vi "APC_HRL.vi"(0 "Pcyl":dbl[][](array[numeric])=array1x7200[7200 elements], 1 "exhaust pressure":dbl[][](array[numeric])=array1x7200[7200 elements], 2 "FilterCoefs":T3={"IIR LowPass"={"filter structure"=enum."IIR 2nd Order", "Reverse Coefficients"=[-1.7786317778245848, 0.8008026466657077], "Forward Coefficients"=[0.005542717210280682, 0.011085434420561363, 0.005542717210280682]}, "IIR HighPass"={"filter structure"=enum."IIR 2nd Order", "Reverse Coefficients"=[], "Forward Coefficients"=[]}} {"IIR LowPass"."Forward Coefficients" format="%.4f"; "IIR LowPass"."Reverse Coefficients" format="%.4f"}, 3 "Expected IMEP":dbl) -> (4 "LPfilt Pcyl":dbl[][](array[numeric]), 5 "HRL [J]":dbl[][](array[numeric]), 6 "CombustionAnalysisCluster":T2={"IMEPn [bar]"=[nan, nan, nan, nan, nan, nan], "IMEPg [bar]"=[nan, nan, nan, nan, nan, nan], "MAPO [bar/CAD]"=[nan, nan, nan, nan, nan, nan], "maxQ [J]"=[nan, nan, nan, nan, nan, nan], "CA10  [CADATDC]"=[nan, nan, nan, nan, nan, nan], "CA50 [CADATDC]"=[nan, nan, nan, nan, nan, nan], "CA90 [CADATDC]"=[nan, nan, nan, nan, nan, nan], "Pmax [bar]"=[nan, nan, nan, nan, nan, nan], "IMEPstd [bar]"=[nan, nan, nan, nan, nan, nan], "CA03  [CADATDC]"=[nan, nan, nan, nan, nan, nan], "CA97  [CADATDC]"=[nan, nan, nan, nan, nan, nan], "CA10CA90 [CADATDC]"=[nan, nan, nan, nan, nan, nan], "maxdpdCAD [bar/CAD]"=[nan, nan, nan, nan, nan, nan], "kappa_comp [-]"=[nan, nan, nan, nan, nan, nan], "kappa_exp [-]"=[nan, nan, nan, nan, nan, nan], "PMEP [bar]"=[nan, nan, nan, nan, nan, nan], "RI [-]"=[nan, nan, nan, nan, nan, nan]}, 7 "HPfilt Pcyl":dbl[][](array[numeric]), 8 "PcylDiagWarningsAndErrors":T1[](array[typedef]))   [LabVIEW 2020]
uses:
  controls/APC_CombustionMetrics.ctl
  controls/APC_PcylDiag.ctl
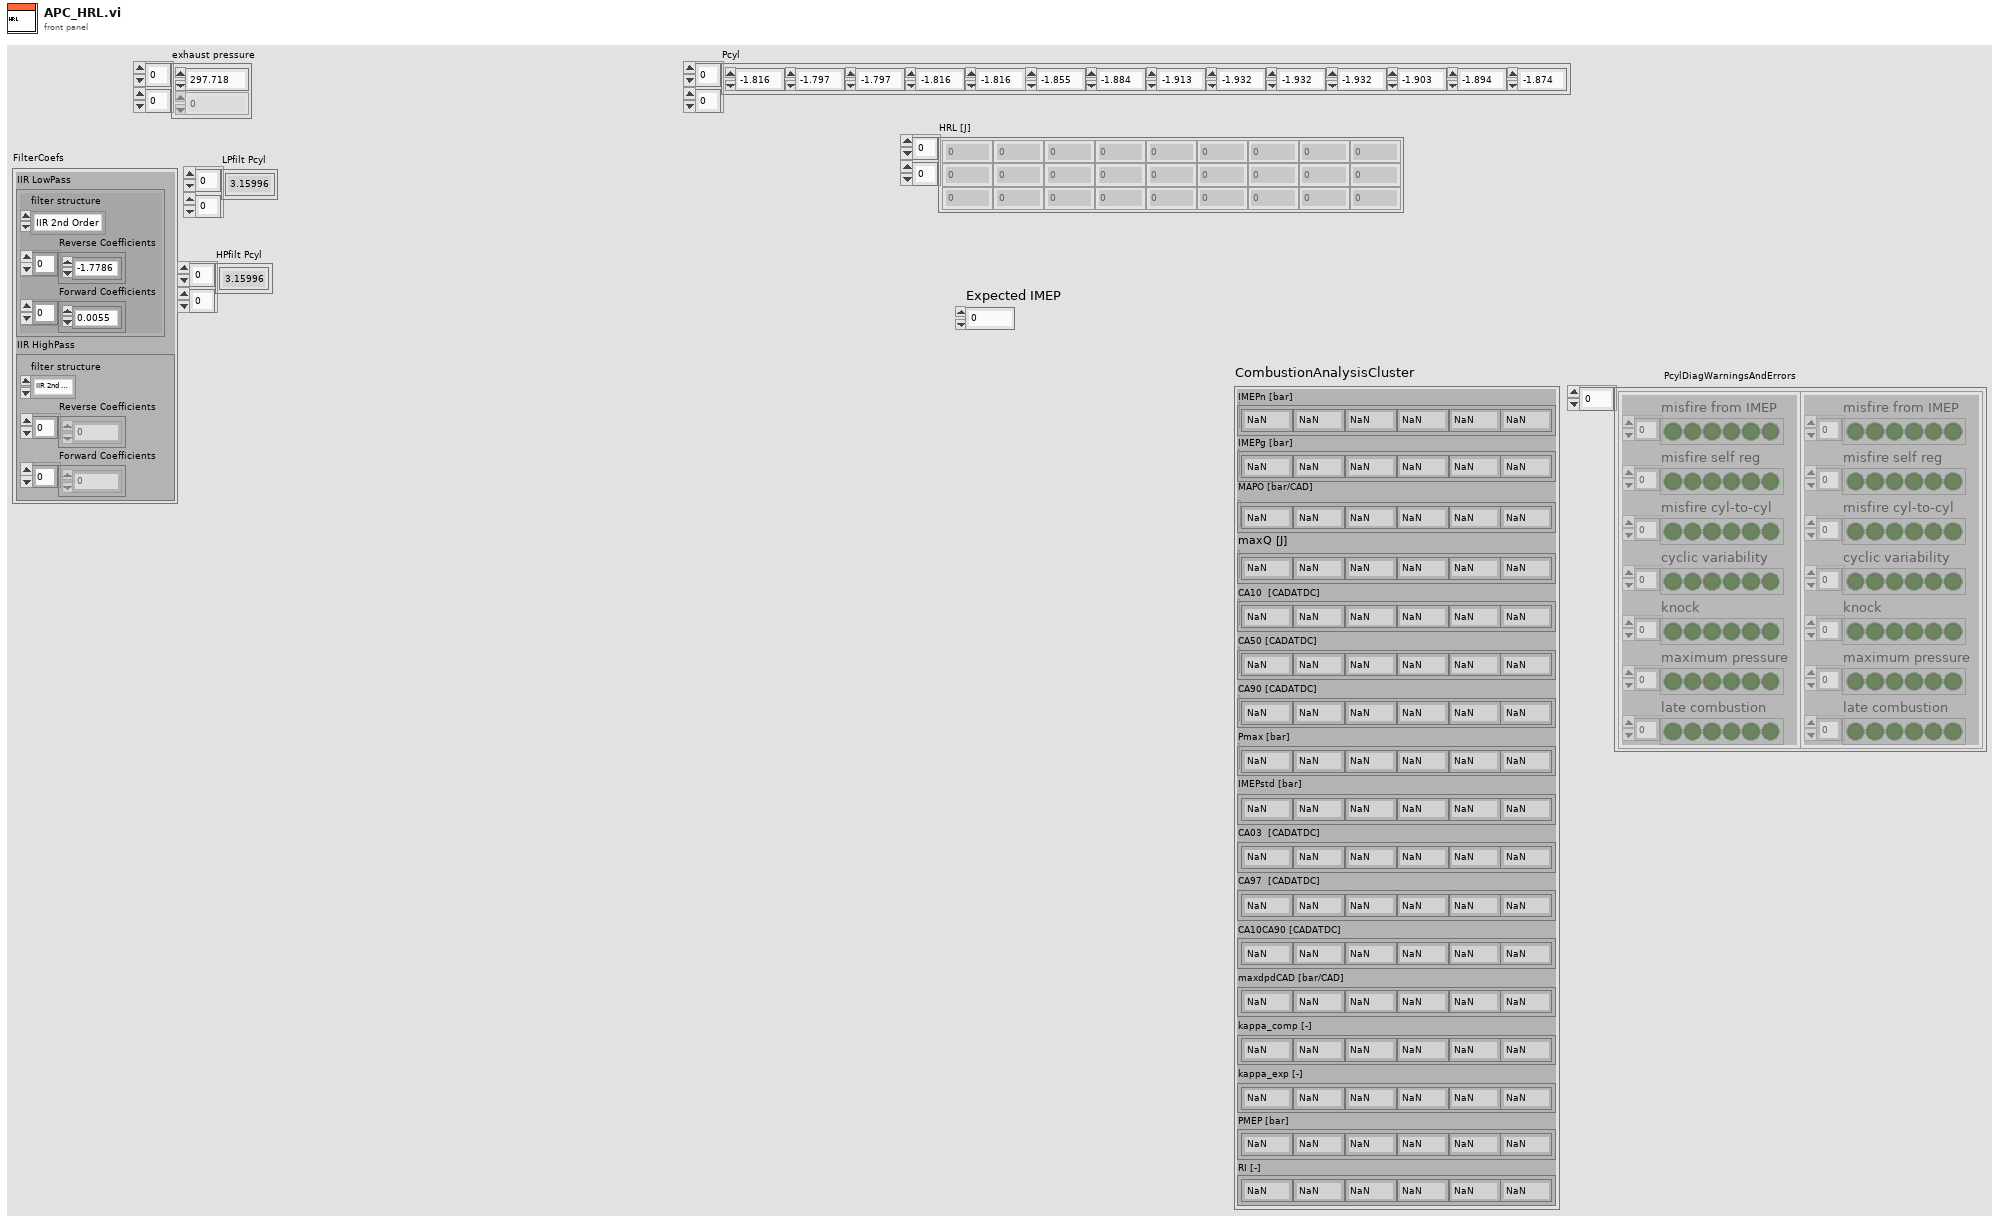
[diagram p1: front panel]
types:
  T1 = typedef "APC_PcylDiag.ctl" = cluster{"misfire from IMEP":bool[], "misfire self reg":bool[], "misfire cyl-to-cyl":bool[], "cyclic variability":bool[], "knock":bool[], "maximum pressure":bool[], "late combustion":bool[]}
  T2 = typedef "APC_CombustionMetrics.ctl" = cluster{"IMEPn [bar]":dbl[], "IMEPg [bar]":dbl[], "MAPO [bar/CAD]":dbl[], "maxQ [J]":dbl[], "CA10  [CADATDC]":dbl[], "CA50 [CADATDC]":dbl[], "CA90 [CADATDC]":dbl[], "Pmax [bar]":dbl[], "IMEPstd [bar]":dbl[], "CA03  [CADATDC]":dbl[], "CA97  [CADATDC]":dbl[], "CA10CA90 [CADATDC]":dbl[], "maxdpdCAD [bar/CAD]":dbl[], "kappa_comp [-]":dbl[], "kappa_exp [-]":dbl[], "PMEP [bar]":dbl[], "RI [-]":dbl[]}
  T3 = cluster{"IIR LowPass":cluster{"filter structure":enum32{"IIR 2nd Order", "IIR 4th Order"}, "Reverse Coefficients":dbl[], "Forward Coefficients":dbl[]}, "IIR HighPass":cluster{"filter structure":enum32{"IIR 2nd Order", "IIR 4th Order"}, "Reverse Coefficients":dbl[], "Forward Coefficients":dbl[]}}
  T4 = cluster{"filter structure":enum32{"IIR 2nd Order", "IIR 4th Order"}, "Reverse Coefficients":dbl[], "Forward Coefficients":dbl[]}
  T5 = typedef "APC_volume.ctl" = cluster{"V [m^3]":dbl[], "dV [m^3/CAD]":dbl[], "Vdis [m^3]":dbl, "Surface [m^2]":dbl[], "CAD/sample":dbl}
  T6 = typedef "APC_CylMetrics.ctl" = cluster{"maxdPdCAD [bar/CAD]":dbl, "kappa_comp":dbl, "kappa_exp":dbl, "maxQ [J]":dbl, "CA03":dbl, "CA10":dbl, "CA50":dbl, "CA90":dbl, "CA97":dbl, "CA10CA90":dbl}
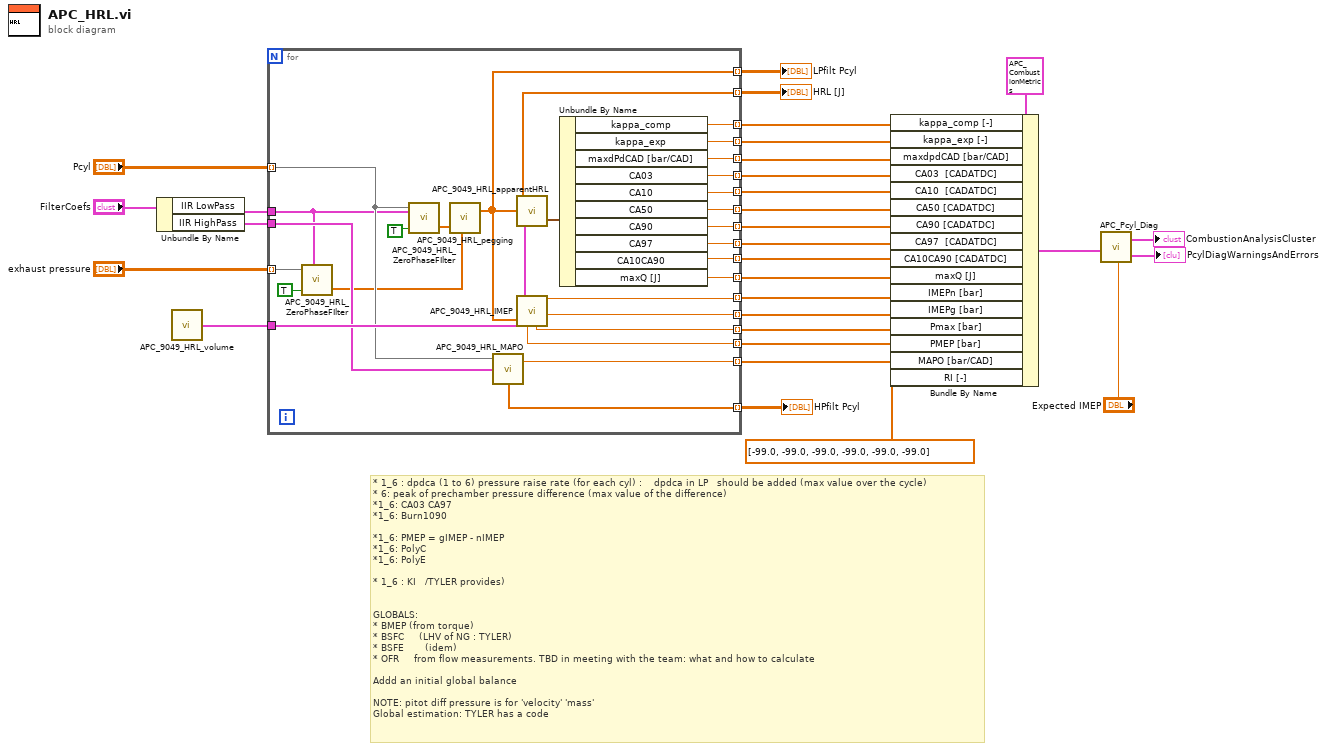
[diagram p0: block diagram]
diagram:
  # "* 1_6 : dpdca (1 to 6) pressure raise rate (for each cyl) :    dpdca in LP   should be added (max value over the cycle)\n* 6: peak of prechamber pressure difference (max value of the difference)\n*1_6: CA03 CA97\n*1_6: Burn1090\n\n*1_6: PMEP = gIMEP - nIMEP\n*1_6: PolyC\n*1_6: PolyE\n\n* 1_6 : KI   /TYLER provides)\n \n\nGLOBALS:\n* BMEP (from torque)\n* BSFC     (LHV of NG : TYLER)\n* BSFE       (idem)\n* OFR     from flow measurements. TBD in meeting with the team: what and how to calculate\n\nAddd an initial global balance \n\nNOTE: pitot diff pressure is for 'velocity' 'mass'\nGlobal estimation: TYLER has a code"
  n1 = Unbundle By Name("FilterCoefs") -> ("IIR LowPass"=w27:T4, "IIR HighPass"=w26:T4)
  n2 = call "APC_9049_HRL_volume.vi"() -> ("Volume cluster"=w30:T5)  [unwired: 2 in]
  n3 = for {
    tunnel: w27 -> [w48]
    tunnel: w30 -> [w57]
    tunnel: "Pcyl" -> [w50] mode=indexing
    tunnel: [w45] -> w29 mode=indexing
    tunnel: [w56] -> w20 mode=indexing
    tunnel: [w55] -> w22 mode=indexing
    tunnel: [w54] -> w25 mode=indexing
    tunnel: w26 -> [w52]
    tunnel: [w51] -> w17 mode=indexing
    tunnel: "exhaust pressure" -> [w47] mode=indexing
    tunnel: [w39] -> w21 mode=indexing
    tunnel: [w34] -> w7 mode=indexing
    tunnel: [w38] -> w10 mode=indexing
    tunnel: [w44] -> w18 mode=indexing
    tunnel: [w43] -> w16 mode=indexing
    tunnel: [w37] -> w15 mode=indexing
    tunnel: [w36] -> w9 mode=indexing
    tunnel: [w40] -> w8 mode=indexing
    tunnel: [w35] -> w6 mode=indexing
    tunnel: [w41] -> w5 mode=indexing
    tunnel: [w33] -> w4 mode=indexing
    tunnel: [w32] -> w3 mode=indexing
    tunnel: [w31] -> w2 mode=indexing
    n4 = call "APC_9049_HRL_ZeroPhaseFIlter.vi"("Init value compensation"=TRUE, "IIR Filter Cluster"=w48, "Pcyl"=w47) -> ("Pcylfilt"=w46:dbl[])  [unwired: 1 out]
    n5 = call "APC_9049_HRL_ZeroPhaseFIlter.vi"("Init value compensation"=TRUE, "IIR Filter Cluster"=w48, "Pcyl"=w50) -> ("Pcylfilt"=w58:dbl[])  [unwired: 1 out]
    n6 = call "APC_9049_HRL_pegging.vi"("exhaust pressure"=w46, "Pcylfilt"=w58) -> ("Pegged Pressure"=w54:dbl[])  [unwired: 1 out]
    n7 = call "APC_9049_HRL_MAPO.vi"("IIR Filter Cluster"=w52, "Pcyl"=w50) -> ("PcylHPfilt"=w43:dbl[], "MAPO"=w51:dbl)  [unwired: 1 in]
    n8 = call "APC_9049_HRL_apparentHRL.vi"("Volume cluster"=w57, "Pegged pressure [bar]"=w54) -> ("CylMetrics"=w42:T6, "HRL [J]"=w45:dbl[])
    n9 = call "APC_9049_HRL_IMEP.vi"("Volume cluster"=w57, "Pressure"=w54) -> ("IMPEn"=w56:dbl, "IMEPg"=w55:dbl, "Pmax"=w44:dbl, "PMEP"=w31:dbl)
    n10 = Unbundle By Name(w42) -> ("kappa_comp"=w33:dbl, "kappa_exp"=w32:dbl, "maxdPdCAD [bar/CAD]"=w41:dbl, "CA03"=w40:dbl, "CA10"=w39:dbl, "CA50"=w38:dbl, "CA90"=w37:dbl, "CA97"=w36:dbl, "CA10CA90"=w35:dbl, "maxQ [J]"=w34:dbl)
  }
  "HRL [J]" <- w29
  "LPfilt Pcyl" <- w25
  "HPfilt Pcyl" <- w16
  n11 = Bundle By Name(cluster=T2 {"IMEPn [bar]"=[nan, nan, nan, nan, nan, nan], "IMEPg [bar]"=[nan, nan, nan, nan, nan, nan], "MAPO [bar/CAD]"=[nan, nan, nan, nan, nan, nan], "maxQ [J]"=[nan, nan, nan, nan, nan, nan], "CA10  [CADATDC]"=[nan, nan, nan, nan, nan, nan], "CA50 [CADATDC]"=[nan, nan, nan, nan, nan, nan], "CA90 [CADATDC]"=[nan, nan, nan, nan, nan, nan], "Pmax [bar]"=[nan, nan, nan, nan, nan, nan], "IMEPstd [bar]"=[nan, nan, nan, nan, nan, nan], "CA03  [CADATDC]"=[nan, nan, nan, nan, nan, nan], "CA97  [CADATDC]"=[nan, nan, nan, nan, nan, nan], "CA10CA90 [CADATDC]"=[nan, nan, nan, nan, nan, nan], "maxdpdCAD [bar/CAD]"=[nan, nan, nan, nan, nan, nan], "kappa_comp [-]"=[nan, nan, nan, nan, nan, nan], "kappa_exp [-]"=[nan, nan, nan, nan, nan, nan], "PMEP [bar]"=[nan, nan, nan, nan, nan, nan], "RI [-]"=[nan, nan, nan, nan, nan, nan]} ("CombustionAnalysisCluster 2"), "kappa_comp [-]"=w4, "kappa_exp [-]"=w3, "maxdpdCAD [bar/CAD]"=w5, "CA03  [CADATDC]"=w8, "CA10  [CADATDC]"=w21, "CA50 [CADATDC]"=w10, "CA90 [CADATDC]"=w15, "CA97  [CADATDC]"=w9, "CA10CA90 [CADATDC]"=w6, "maxQ [J]"=w7, "IMEPn [bar]"=w20, "IMEPg [bar]"=w22, "Pmax [bar]"=w18, "PMEP [bar]"=w2, "MAPO [bar/CAD]"=w17, "RI [-]"=dbl[] [-99.0, -99.0, -99.0, -99.0, -99.0, -99.0]) -> (w14:T2)
  n12 = call "APC_Pcyl_Diag.vi"("Expected IMEP"="Expected IMEP", "CombustionAnalysisCluster"=w14) -> ("WarningsAndErrors"=→"PcylDiagWarningsAndErrors":T1[], "CombustionAnalysisClusterOut"=→"CombustionAnalysisCluster":T2)
